vi "Read (Multiple Points).vi"(0 "VISA resource name":refnum<visa-resource-name>, 1 "Timeout (10000 ms)":i32=10000, 5 "Buffer Name (\"\")":string, 7 "Capture Mode(0: Scan)":i32(ring) items=["Scan", "Trigger"], 9 "Clear Buffer (No)":bool, 11 "error in (no error)":errorcluster, 12 "Buffer Element1 ()":i32(ring) items=["", "Date", "Extra", "Formatted", "Fractional", "Reading", "Relative", "Seconds", "Status", "Time", "Tstamp", "Unit", "CHAN", "Extra Format", "Extra Unit"], 13 "Buffer Element2 ()":i32(ring) items=["", "Date", "Extra", "Formatted", "Fractional", "Reading", "Relative", "Seconds", "Status", "Time", "Tstamp", "Unit", "CHAN", "Extra Form", "Extra Unit"]) -> (4 "VISA resource name out":refnum<visa-resource-name>, 6 "Measurements":dbl[](array[numeric]), 15 "error out":errorcluster)   [LabVIEW 2016, in "Keithley DMM6500 DAQ6500 Series.lvlib"]
doc: "Reads and returns multiple measurements from the instrument. Use this VI when you want to take multiple measurements using an immediate trigger. Use the low-level VIs for other triggering options."
uses:
  Keithley DMM6500 DAQ6500 Series.lvlib
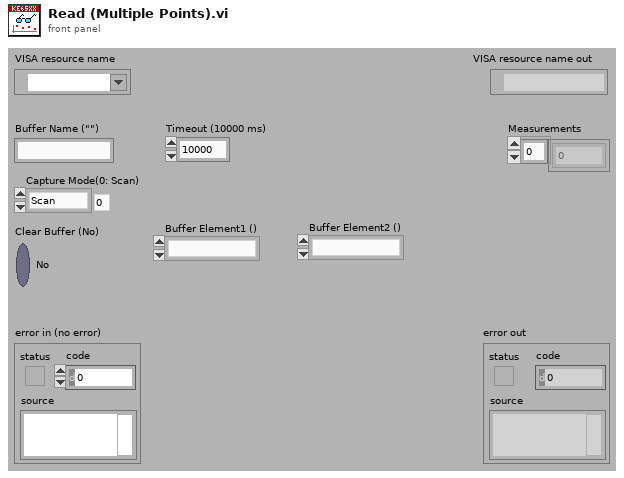
[diagram p1: front panel]
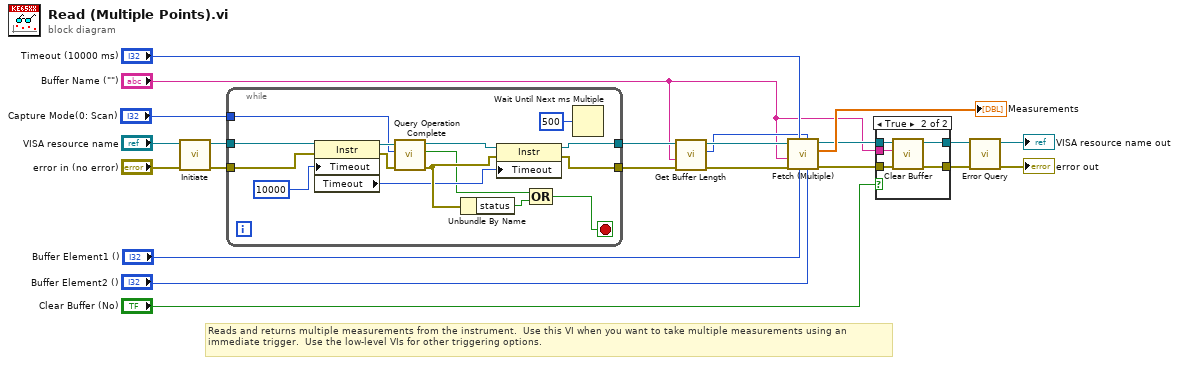
[diagram p0: block diagram]
diagram:
  # "Reads and returns multiple measurements from the instrument.  Use this VI when you want to take multiple measurements using an immediate trigger.  Use the low-level VIs for other triggering options."
  n1 = call "Initiate.vi"("error in (no error)"="error in (no error)", "VISA resource name"="VISA resource name") -> ("error out"=w14:errorcluster, "VISA resource name out"=w15:refnum<visa-resource-name>)  [unwired: 8 in]
  n2 = while {
    tunnel: w15 -> [w34]
    tunnel: w14 -> [w33]
    tunnel: [w30] -> w11
    tunnel: [w29] -> w10
    tunnel: "Capture Mode(0: Scan)" -> [w23]
    stop <- w36 stop-if-true
    n3 = property on="Property Node" class="Instr"(reference=w34, error in=w33, "Timeout"=u32 10000 ("General Settings:Timeout Value")) -> (reference out=w32:refnum<visa-resource-name>, error out=w31:errorcluster, "Timeout"=w26:u32)
    n4 = call "Query Operation Complete.vi"("error in (no error)"=w31, "Capture Mode (0: Scan)"=w23, "VISA resource name"=w32) -> ("error out"=w27:errorcluster, "Complete"=w24:bool, "VISA resource name out"=w28:refnum<visa-resource-name>)  [unwired: 6 in]
    n5 = Unbundle By Name(w27) -> ("status"=w35:bool)
    n6 = property on="Property Node" class="Instr"(reference=w28, error in=w27, "Timeout"=w26) -> (reference out=w30:refnum<visa-resource-name>, error out=w29:errorcluster)
    n7 = Compound Arithmetic op=OR(w24, w35) -> (w36:bool)
    n8 = Wait Until Next ms Multiple(millisecond multiple=u32 500) -> ()  [unwired: 1 out]
  }
  n9 = call "Get Buffer Length.vi"("error in (no error)"=w10, "Buffer Name ()"="Buffer Name (\"\")", "VISA resource name"=w11) -> ("error out"=w12:errorcluster, "Buffer Count"=w9:i32, "VISA resource name out"=w13:refnum<visa-resource-name>)  [unwired: 6 in]
  n10 = call "Fetch (Multiple).vi"("Buffer Element2 ()"="Buffer Element2 ()", "Sample Count (0)"=w9, "Buffer Element1 ()"="Buffer Element1 ()", "Timeout (100000 ms)"="Timeout (10000 ms)", "error in (no error)"=w12, "Buffer Name ()"="Buffer Name (\"\")", "VISA resource name"=w13) -> ("error out"=w17:errorcluster, "Measurements"=→"Measurements":dbl[], "VISA resource name out"=w18:refnum<visa-resource-name>)  [unwired: 2 in]
  n11 = case shown="True" "Clear Buffer (No)" {
    tunnel: [w39 w44] -> w6
    tunnel: [w38 w43] -> w5
    tunnel: w18 -> [w39 w42]
    tunnel: w17 -> [w38 w41]
    tunnel: "Buffer Name (\"\")" -> [_ w40]
    frame False {
    }
    frame True {
      n12 = call "Clear Buffer.vi"("error in (no error)"=w41, "Buffer Name (\"\")"=w40, "VISA resource name"=w42) -> ("error out"=w43:errorcluster, "VISA resource name out"=w44:refnum<visa-resource-name>)  [unwired: 7 in]
    }
  }
  n13 = call "Error Query.vi"("error in (no error)"=w5, "VISA resource name"=w6) -> ("error out"=→"error out":errorcluster, "VISA resource name out"=→"VISA resource name out":refnum<visa-resource-name>)  [unwired: 6 in, 2 out]
